vi "Hopper Position Variable.vi"() -> ()   [LabVIEW 2019]
panel:
  in  "Hopper Position":string="10\n10"
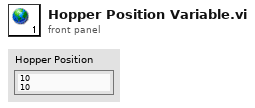
[diagram p1: front panel]
diagram:
